vi "IO.vi"() -> ()   [LabVIEW 2020]
uses:
  Global_Variable/Global.vi
  Libraries/S7/S7.lvlib
panel:
  in  "选项卡控件":enum32{"DI", "DO", "伺服"}(tab)
  out "I 1":T1
  out "I 3":T2
  out "I 2":T3
  out "I 0":T4
  out "I 4":T5
  out "I 5":T6
  in  "Q5":T7
  in  "Q4":T8
  in  "Q3":T9
  in  "Q2":T10
  in  "Q1":T11
  in  "Q0":T12
  in  "工位一系数":dbl=1.0
  in  "工位二系数":dbl=1.0
  out "工位一编码器位移":sgl caption="工位一编码器" format="%#.3f"
  out "工位二编码器位移":sgl caption="工位二编码器" format="%#.3f"
  out "工位一扭矩":sgl format="%#.3f"
  out "工位二扭矩":sgl format="%#.3f"
  in  "工位二移载伺服手动速度":sgl caption="手动速度" format="%#.3f"
  in  "工位二移载伺服-正转":bool
  in  "工位二移载伺服-反转":bool
  in  "工位二移载伺服绝对位置":sgl caption="绝对位置" format="%#.3f"
  in  "工位二移载伺服相对位置":sgl caption="相对位置" format="%#.3f"
  out "工位二移载伺服当前位置":sgl caption="当前位置" format="%#.3f"
  in  "工位二移载伺服-绝对定位":bool
  in  "工位二移载伺服-相对定位":bool
  out "工位二移载伺服状态":bool
  in  "工位一旋转伺服手动速度":sgl caption="手动速度" format="%#.3f"
  in  "工位一旋转伺服-正转":bool
  in  "工位一旋转伺服-反转":bool
  in  "工位一旋转伺服绝对位置":sgl caption="绝对位置" format="%#.3f"
  in  "工位一旋转伺服相对位置":sgl caption="相对位置" format="%#.3f"
  out "工位一驱动伺服当前位置":sgl caption="当前位置" format="%#.3f"
  in  "工位一旋转伺服-绝对定位":bool
  in  "工位一旋转伺服-相对定位":bool
  in  "工位二旋转伺服手动速度":sgl caption="手动速度" format="%#.3f"
  in  "工位二旋转伺服-正转":bool
  in  "工位二旋转伺服-反转":bool
  in  "工位二旋转伺服绝对位置":sgl caption="绝对位置" format="%#.3f"
  in  "工位二旋转伺服相对位置":sgl caption="相对位置" format="%#.3f"
  out "工位二驱动伺服当前位置":sgl caption="当前位置" format="%#.3f"
  in  "工位二旋转伺服-绝对定位":bool
  in  "工位二旋转伺服-相对定位":bool
  in  "工位一移载伺服手动速度":sgl caption="手动速度" format="%#.3f"
  in  "工位一移载伺服-正转":bool
  in  "工位一移载伺服-反转":bool
  in  "工位一移载伺服绝对位置":sgl caption="绝对位置" format="%#.3f"
  in  "工位一移载伺服相对位置":sgl caption="相对位置" format="%#.3f"
  out "工位一移载当前位置":sgl caption="当前位置" format="%#.3f"
  in  "工位一移载伺服-绝对定位":bool
  in  "工位一移载伺服-相对定位":bool
  out "工位一旋转伺服状态":bool
  out "工位二旋转伺服状态":bool
  out "工位一移载伺服状态":bool
  # "手动操作"
  # "工位二移载伺服"
  # "工位一旋转伺服"
  # "工位一移载伺服"
  # "工位二旋转伺服"
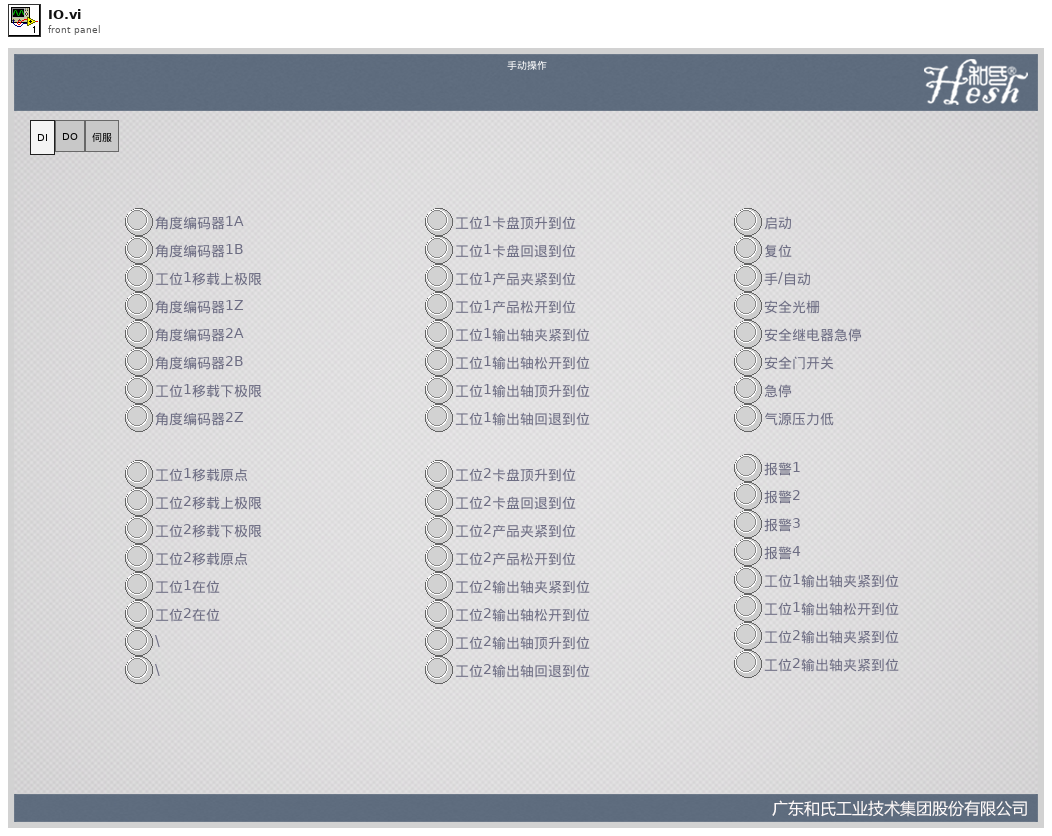
[diagram p1: front panel]
types:
  T1 = cluster{"工位1移载原点":bool, "工位2移载上极限":bool, "工位2移载下极限":bool, "工位2移载原点":bool, "工位1在位":bool, "工位2在位":bool, "\\":bool, "\\ ":bool}
  T2 = cluster{"工位2卡盘顶升到位":bool, "工位2卡盘回退到位":bool, "工位2产品夹紧到位":bool, "工位2产品松开到位":bool, "工位2输出轴夹紧到位":bool, "工位2输出轴松开到位":bool, "工位2输出轴顶升到位":bool, "工位2输出轴回退到位":bool}
  T3 = cluster{"工位1卡盘顶升到位":bool, "工位1卡盘回退到位":bool, "工位1产品夹紧到位":bool, "工位1产品松开到位":bool, "工位1输出轴夹紧到位":bool, "工位1输出轴松开到位":bool, "工位1输出轴顶升到位":bool, "工位1输出轴回退到位":bool}
  T4 = cluster{"角度编码器1A":bool, "角度编码器1B":bool, "工位1移载上极限":bool, "角度编码器1Z":bool, "角度编码器2A":bool, "角度编码器2B":bool, "工位1移载下极限":bool, "角度编码器2Z":bool}
  T5 = cluster{"启动":bool, "复位":bool, "手/自动":bool, "安全光栅":bool, "安全继电器急停":bool, "安全门开关":bool, "急停":bool, "气源压力低":bool}
  T6 = cluster{"报警1":bool, "报警2":bool, "报警3":bool, "报警4":bool, "工位1输出轴夹紧到位":bool, "工位1输出轴松开到位":bool, "工位2输出轴夹紧到位":bool, "工位2输出轴夹紧到位":bool}
  T7 = cluster{"工位1卡盘顶升":bool, "工位1卡盘回退":bool, "工位2卡盘顶升":bool, "工位2卡盘回退":bool, "备用":bool, "备用":bool, "备用":bool, "备用":bool}
  T8 = cluster{"工位1合格指示灯":bool, "工位1不合格指示灯":bool, "工位2合格指示灯":bool, "工位2不合格指示灯":bool, "总气阀":bool, "工位2采集切换":bool, "工位1采集切换":bool, "备用":bool}
  T9 = cluster{"工位2输入轴夹紧":bool, "工位2输入轴松开":bool, "工位2产品夹紧":bool, "工位2产品松开":bool, "工位2输出轴夹紧":bool, "工位2输出轴松开":bool, "工位2输出轴顶升":bool, "工位2输出轴回退":bool}
  T10 = cluster{"工位1输入轴夹紧":bool, "工位1输入轴松开":bool, "工位1产品夹紧":bool, "工位1产品松开":bool, "工位1输出轴夹紧":bool, "工位1输出轴松开":bool, "工位1输出轴顶升":bool, "工位1输出轴回退":bool}
  T11 = cluster{"备用":bool, "备用":bool, "/":bool, "/":bool, "/":bool, "/":bool, "/":bool, "/":bool}
  T12 = cluster{"备用":bool, "备用":bool, "备用":bool, "备用":bool, "三色灯-红":bool, "三色灯-黄":bool, "三色灯-绿":bool, "三色灯-蜂鸣器":bool}
  T13 = cluster{bool, bool, bool, bool, bool, bool, bool, bool}
  T14 = typedef "S7.lvlib/Read_Data (Reply Payload)--cluster.ctl" = cluster{"读取成功":bool, "数据":u32[], "Read_Data_error":errorcluster}
  T15 = cluster{"Boolean array[0]":bool, "Boolean array[1]":bool, "Boolean array[2]":bool, "Boolean array[3]":bool, "Boolean array[4]":bool, "Boolean array[5]":bool, "Boolean array[6]":bool, "Boolean array[7]":bool}
  T16 = cluster{"工位一驱动伺服位移":sgl, "工位二驱动伺服位移":sgl, "工位一移载伺服位移":sgl, "工位二移载伺服位移":sgl, "工位一编码器位移":sgl, "工位二编码器位移":sgl, "工位一扭矩":sgl, "工位二扭矩":sgl}
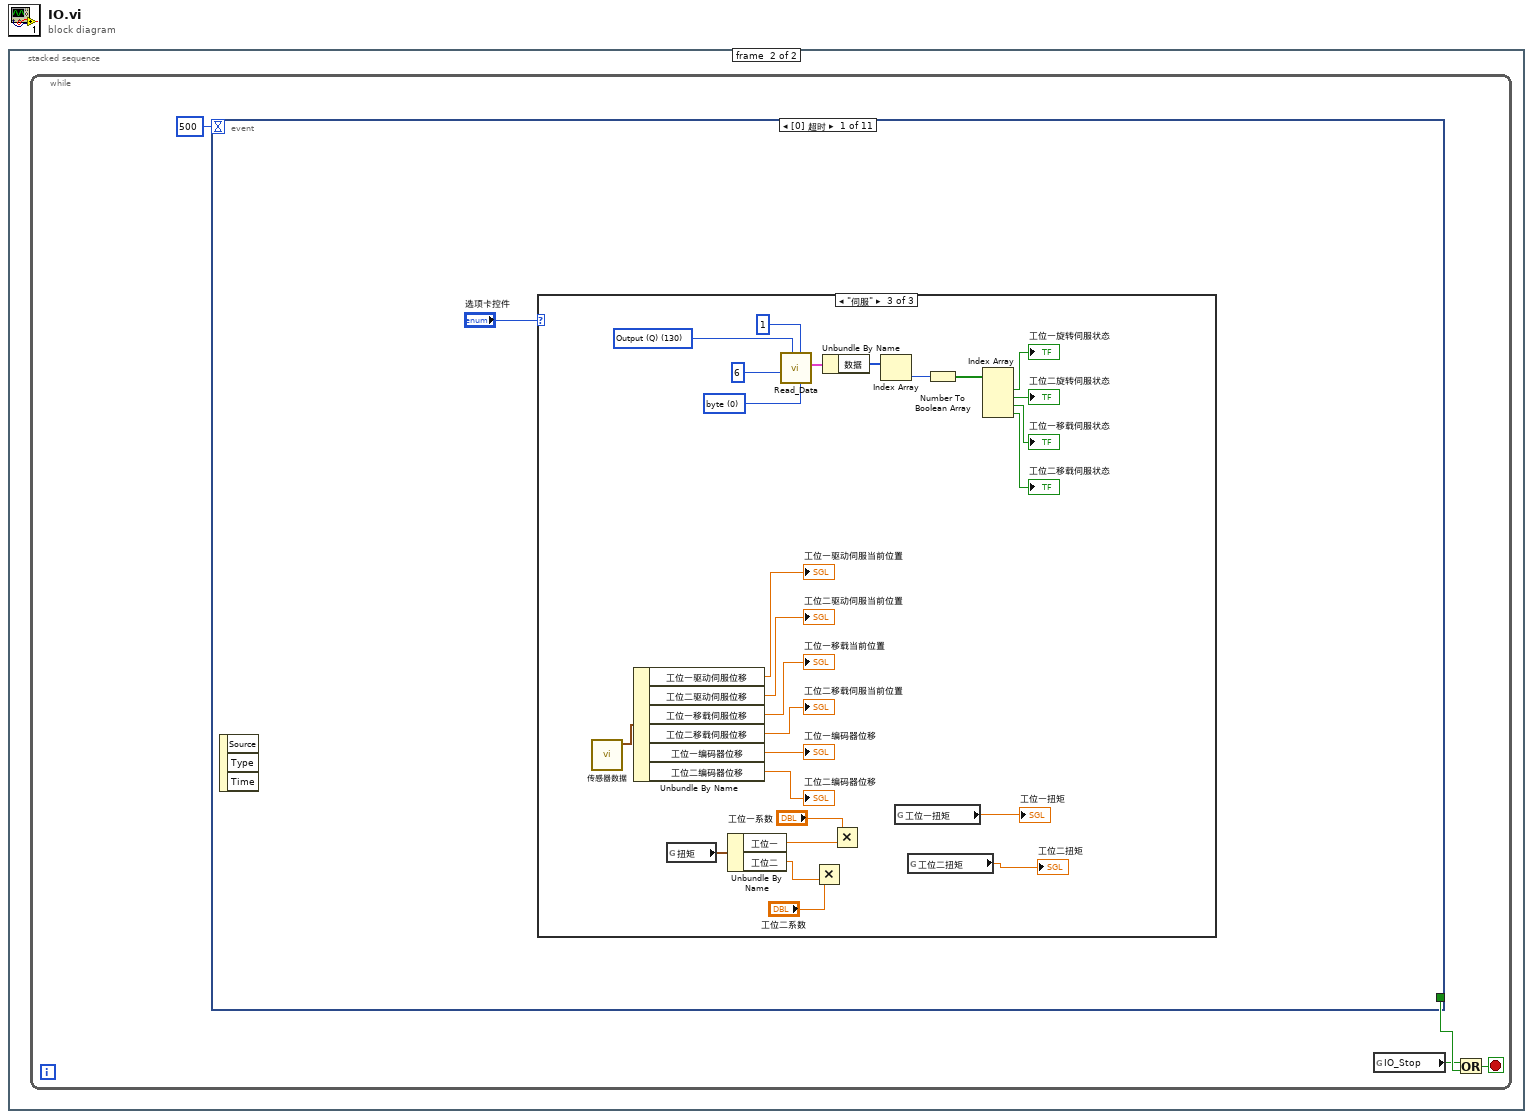
[diagram p0: block diagram]
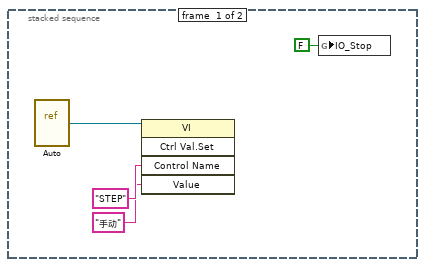
[diagram p2: hidden frame]
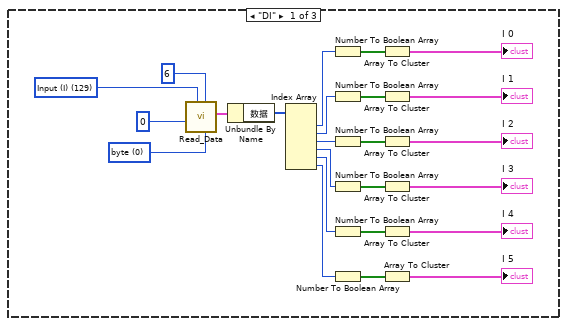
[diagram p3: hidden frame]
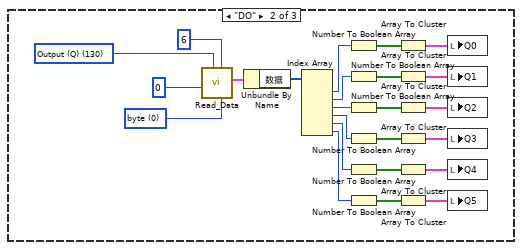
[diagram p4: hidden frame]
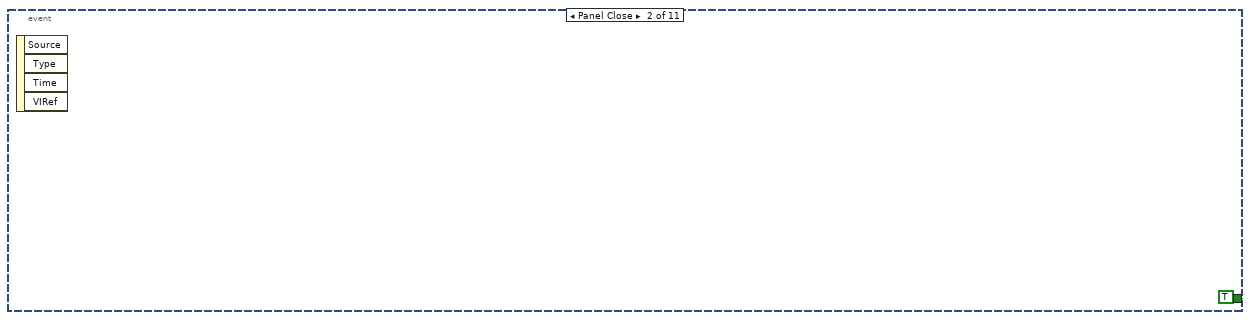
[diagram p5: hidden frame]
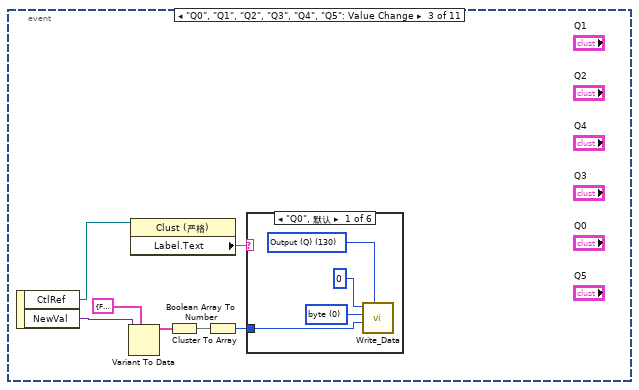
[diagram p6: hidden frame]
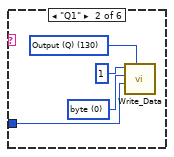
[diagram p7: hidden frame]
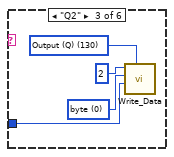
[diagram p8: hidden frame]
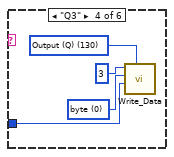
[diagram p9: hidden frame]
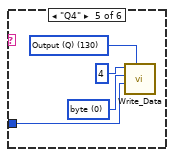
[diagram p10: hidden frame]
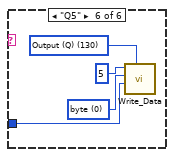
[diagram p11: hidden frame]
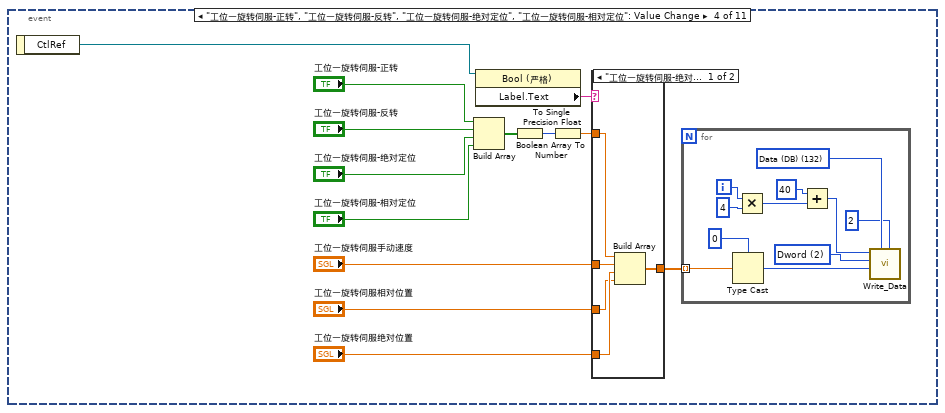
[diagram p12: hidden frame]
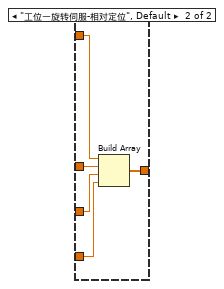
[diagram p13: hidden frame]
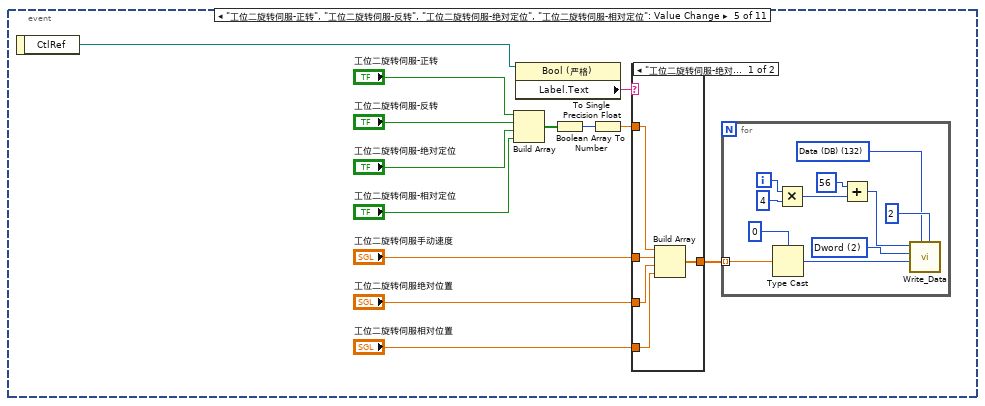
[diagram p14: hidden frame]
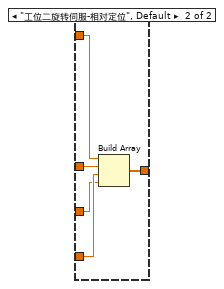
[diagram p15: hidden frame]
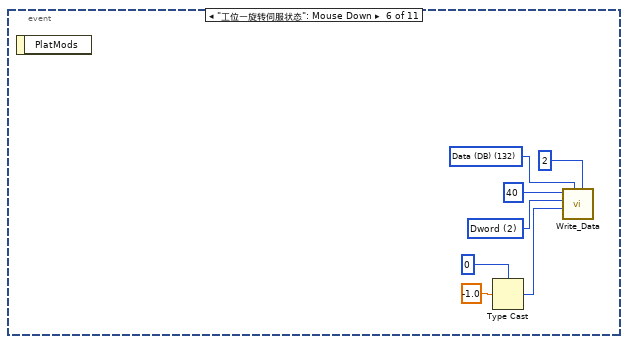
[diagram p16: hidden frame]
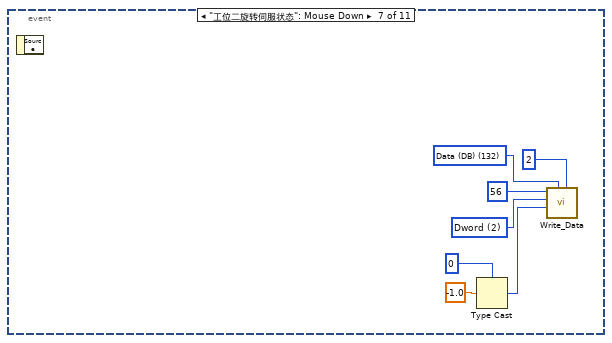
[diagram p17: hidden frame]
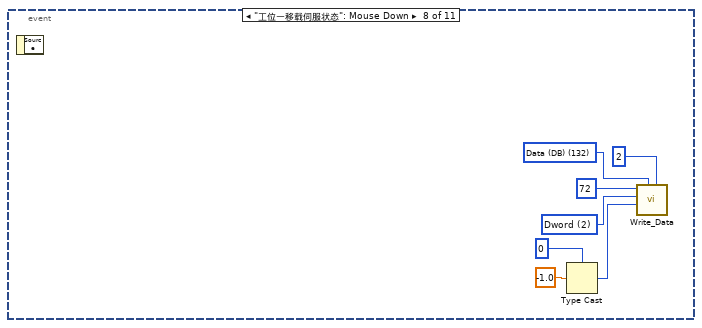
[diagram p18: hidden frame]
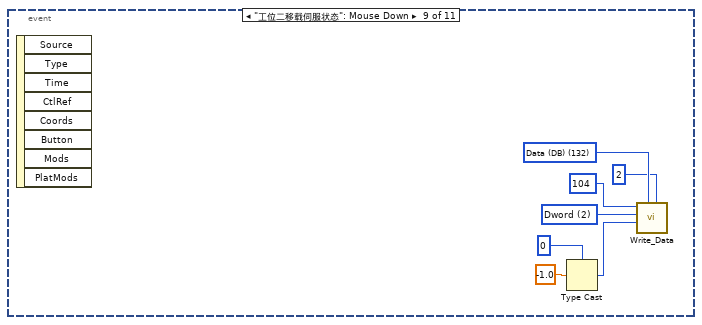
[diagram p19: hidden frame]
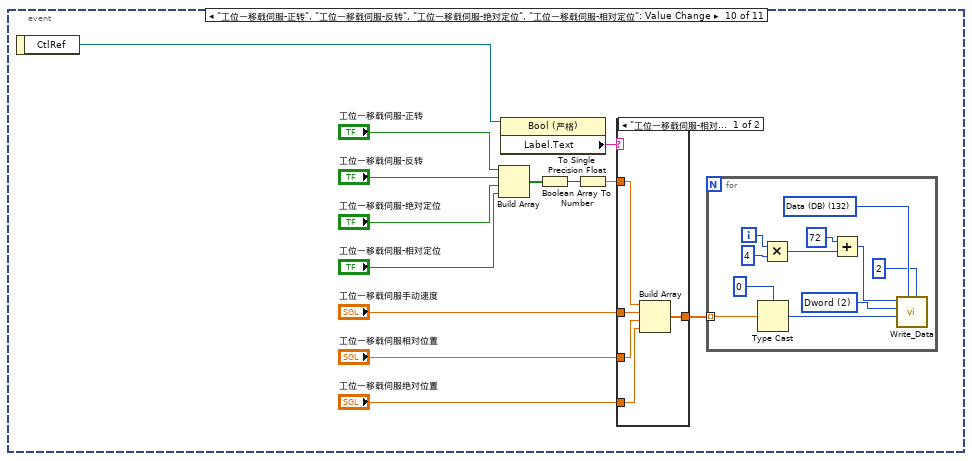
[diagram p20: hidden frame]
diagram:
  n1 = stacked-sequence {
    frame #0 {
      n2 = vi-ref "Auto.vi"() -> (w3:refnum<vi>)
      n3 = invoke class="VI" method="Ctrl Val.Set"(reference=w3, "Control Name"="STEP" ("控件名"), "Value"="手动" ("控件名")) -> ()  [unwired: 2 in, 5 out]
      n4 = global write "Global.vi" "IO_Stop"(FALSE ("IO_Stop")) -> ()
    }
    frame #1 {
      n5 = while {
        stop <- w5 stop-if-true
        n6 = event shown="[0] 超时" {
          selector: _ -> [_ _ _ _ _ _ _ _ _ _ _]
          dyn-events: _ -> [_ _ _ _ _ _ _ _ _ _ _]
          timeout: 500 -> [_ _ _ _ _ _ _ _ _ _ _]
          tunnel: [_ TRUE _ _ _ _ _ _ _ _ _] -> w7
          event Timeout {
            n7 = event-data() -> ()  [unwired: 1 in, 3 out]
            n8 = case shown="\"伺服\"" "选项卡控件" {
              frame "DI" {
                w13 = u16 0 items=["byte", "word", "Dword"] ("数据类型")
                w11 = u8 129 items=["I/O (P)"=128, "Input (I)"=129, "Output (Q)"=130, "Bit Memory (M)"=131, "Data (DB)"=132, "Instance Data (DI)"=133, "Local Data (L)"=134, "Predecessor Local Data (VL)"=135] ("寄存器类型")
                n9 = call "Read_Data.vi"("数据类型"=w13, "读取长度"=u16 6, "寄存器类型"=w11, "起始地址"=u32 0) -> ("Reply Payload"=w15:T14)  [unwired: 5 in, 2 out]
                n10 = Unbundle By Name(w15) -> ("数据"=w14:u32[])
                n11 = Index Array(array=w14) -> (element #1=w27:u32, element #2=w29:u32, element #3=w28:u32, element #4=w24:u32, element #5=w23:u32, element #6=w22:u32)  [unwired: 6 in]
                n12 = Number To Boolean Array(number=w27) -> (Boolean array=w26:bool[])
                n13 = Number To Boolean Array(number=w29) -> (Boolean array=w25:bool[])
                n14 = Number To Boolean Array(number=w28) -> (Boolean array=w21:bool[])
                n15 = Number To Boolean Array(number=w24) -> (Boolean array=w19:bool[])
                n16 = Number To Boolean Array(number=w23) -> (Boolean array=w17:bool[])
                n17 = Number To Boolean Array(number=w22) -> (Boolean array=w16:bool[])
                n18 = Array To Cluster(array=w26) -> (cluster=→"I 0":T15)
                n19 = Array To Cluster(array=w25) -> (cluster=→"I 1":T15)
                n20 = Array To Cluster(array=w21) -> (cluster=→"I 2":T15)
                n21 = Array To Cluster(array=w19) -> (cluster=→"I 3":T15)
                n22 = Array To Cluster(array=w17) -> (cluster=→"I 4":T15)
                n23 = Array To Cluster(array=w16) -> (cluster=→"I 5":T15)
              }
              frame "DO" {
                w37 = u16 0 items=["byte", "word", "Dword"] ("数据类型")
                w35 = u8 130 items=["I/O (P)"=128, "Input (I)"=129, "Output (Q)"=130, "Bit Memory (M)"=131, "Data (DB)"=132, "Instance Data (DI)"=133, "Local Data (L)"=134, "Predecessor Local Data (VL)"=135] ("寄存器类型")
                n24 = call "Read_Data.vi"("数据类型"=w37, "读取长度"=u16 6, "寄存器类型"=w35, "起始地址"=u32 0) -> ("Reply Payload"=w56:T14)  [unwired: 5 in, 2 out]
                n25 = Unbundle By Name(w56) -> ("数据"=w57:u32[])
                n26 = Index Array(array=w57) -> (element #1=w47:u32, element #2=w49:u32, element #3=w48:u32, element #4=w46:u32, element #5=w45:u32, element #6=w44:u32)  [unwired: 6 in]
                n27 = Number To Boolean Array(number=w47) -> (Boolean array=w50:bool[])
                n28 = Number To Boolean Array(number=w49) -> (Boolean array=w51:bool[])
                n29 = Number To Boolean Array(number=w48) -> (Boolean array=w52:bool[])
                n30 = Number To Boolean Array(number=w46) -> (Boolean array=w53:bool[])
                n31 = Number To Boolean Array(number=w45) -> (Boolean array=w54:bool[])
                n32 = Number To Boolean Array(number=w44) -> (Boolean array=w55:bool[])
                n33 = Array To Cluster(array=w50) -> (cluster=w42:T15)
                n34 = Array To Cluster(array=w51) -> (cluster=w43:T15)
                n35 = Array To Cluster(array=w52) -> (cluster=w40:T15)
                n36 = Array To Cluster(array=w53) -> (cluster=w41:T15)
                n37 = Array To Cluster(array=w54) -> (cluster=w39:T15)
                n38 = Array To Cluster(array=w55) -> (cluster=w38:T15)
                n39 = local write "Q0"(w42) -> ()
                n40 = local write "Q1"(w43) -> ()
                n41 = local write "Q2"(w40) -> ()
                n42 = local write "Q3"(w41) -> ()
                n43 = local write "Q4"(w39) -> ()
                n44 = local write "Q5"(w38) -> ()
              }
              frame "伺服" {
                w76 = u16 0 items=["byte", "word", "Dword"] ("数据类型")
                w74 = u8 130 items=["I/O (P)"=128, "Input (I)"=129, "Output (Q)"=130, "Bit Memory (M)"=131, "Data (DB)"=132, "Instance Data (DI)"=133, "Local Data (L)"=134, "Predecessor Local Data (VL)"=135] ("寄存器类型")
                n45 = call "传感器数据.vi"() -> ("传感器读数"=w72:T16)  [unwired: 11 in]
                n46 = Unbundle By Name(w72) -> ("工位一驱动伺服位移"=→"工位一驱动伺服当前位置":sgl, "工位二驱动伺服位移"=→"工位二驱动伺服当前位置":sgl, "工位一移载伺服位移"=→"工位一移载当前位置":sgl, "工位二移载伺服位移"=→"工位二移载伺服当前位置":sgl, "工位一编码器位移"=→"工位一编码器位移":sgl, "工位二编码器位移"=→"工位二编码器位移":sgl)
                n47 = global read "Global.vi" "扭矩"() -> (w64:cluster{"工位一":dbl, "工位二":dbl})
                n48 = Unbundle By Name(w64) -> ("工位一"=w63:dbl, "工位二"=w62:dbl)
                n49 = call "Read_Data.vi"("数据类型"=w76, "读取长度"=u16 1, "寄存器类型"=w74, "起始地址"=u32 6) -> ("Reply Payload"=w77:T14)  [unwired: 5 in, 2 out]
                n50 = Multiply(x="工位二系数", y=w62) -> ()  [unwired: 1 out]
                n51 = Unbundle By Name(w77) -> ("数据"=w78:u32[])
                n52 = Multiply(x="工位一系数", y=w63) -> ()  [unwired: 1 out]
                n53 = Index Array(array=w78) -> (element=w83:u32)  [unwired: 1 in]
                n54 = global read "Global.vi" "工位一扭矩"() -> (→"工位一扭矩":dbl)
                n55 = global read "Global.vi" "工位二扭矩"() -> (→"工位二扭矩":dbl)
                n56 = Number To Boolean Array(number=w83) -> (Boolean array=w80:bool[])
                n57 = Index Array(array=w80) -> (element #1=→"工位一旋转伺服状态":bool, element #2=→"工位二旋转伺服状态":bool, element #3=→"工位一移载伺服状态":bool, element #4=→"工位二移载伺服状态":bool)  [unwired: 4 in]
              }
            }
          }
          event Panel Close {
            n58 = event-data() -> ()  [unwired: 1 in, 4 out]
          }
          event "Q0", "Q1", "Q2", "Q3", "Q4", "Q5": Value Change {
            n59 = event-data() -> ("CtlRef"=w86:refnum<vi>, "NewVal"=w90:variant)  [unwired: 1 in]
            n60 = Variant To Data(type=T13 {FALSE, FALSE, FALSE, FALSE, FALSE, FALSE, FALSE, FALSE}, Variant=w90) -> (data=w89:T13)  [unwired: 1 in, 1 out]
            n61 = property class="Clust (严格)"(reference=w86) -> ("Label.Text"=w85:string)  [unwired: 1 in, 2 out]
            n62 = Cluster To Array(cluster=w89) -> (array=w88:bool[])
            n63 = Boolean Array To Number(Boolean array=w88) -> (number=w87:u32)
            n64 = case shown="\"Q0\", 默认" w85 {
              tunnel: w87 -> [w95 w99 w103 w107 w111 w115]
              frame "Q0", Default {
                w93 = u16 0 items=["byte", "word", "Dword"] ("数据类型")
                w94 = u8 130 items=["I/O (P)"=128, "Input (I)"=129, "Output (Q)"=130, "Bit Memory (M)"=131, "Data (DB)"=132, "Instance Data (DI)"=133, "Local Data (L)"=134, "Predecessor Local Data (VL)"=135] ("寄存器类型")
                n65 = call "Write_Data.vi"("寄存器类型"=w94, "写入数据"=w95, "数据类型"=w93, "写入地址"=u32 0) -> ()  [unwired: 5 in, 3 out]
              }
              frame "Q1" {
                w97 = u16 0 items=["byte", "word", "Dword"] ("数据类型")
                w98 = u8 130 items=["I/O (P)"=128, "Input (I)"=129, "Output (Q)"=130, "Bit Memory (M)"=131, "Data (DB)"=132, "Instance Data (DI)"=133, "Local Data (L)"=134, "Predecessor Local Data (VL)"=135] ("寄存器类型")
                n66 = call "Write_Data.vi"("寄存器类型"=w98, "写入数据"=w99, "数据类型"=w97, "写入地址"=u32 1) -> ()  [unwired: 5 in, 3 out]
              }
              frame "Q2" {
                w101 = u16 0 items=["byte", "word", "Dword"] ("数据类型")
                w102 = u8 130 items=["I/O (P)"=128, "Input (I)"=129, "Output (Q)"=130, "Bit Memory (M)"=131, "Data (DB)"=132, "Instance Data (DI)"=133, "Local Data (L)"=134, "Predecessor Local Data (VL)"=135] ("寄存器类型")
                n67 = call "Write_Data.vi"("寄存器类型"=w102, "写入数据"=w103, "数据类型"=w101, "写入地址"=u32 2) -> ()  [unwired: 5 in, 3 out]
              }
              frame "Q3" {
                w105 = u16 0 items=["byte", "word", "Dword"] ("数据类型")
                w106 = u8 130 items=["I/O (P)"=128, "Input (I)"=129, "Output (Q)"=130, "Bit Memory (M)"=131, "Data (DB)"=132, "Instance Data (DI)"=133, "Local Data (L)"=134, "Predecessor Local Data (VL)"=135] ("寄存器类型")
                n68 = call "Write_Data.vi"("寄存器类型"=w106, "写入数据"=w107, "数据类型"=w105, "写入地址"=u32 3) -> ()  [unwired: 5 in, 3 out]
              }
              frame "Q4" {
                w109 = u16 0 items=["byte", "word", "Dword"] ("数据类型")
                w110 = u8 130 items=["I/O (P)"=128, "Input (I)"=129, "Output (Q)"=130, "Bit Memory (M)"=131, "Data (DB)"=132, "Instance Data (DI)"=133, "Local Data (L)"=134, "Predecessor Local Data (VL)"=135] ("寄存器类型")
                n69 = call "Write_Data.vi"("寄存器类型"=w110, "写入数据"=w111, "数据类型"=w109, "写入地址"=u32 4) -> ()  [unwired: 5 in, 3 out]
              }
              frame "Q5" {
                w113 = u16 0 items=["byte", "word", "Dword"] ("数据类型")
                w114 = u8 130 items=["I/O (P)"=128, "Input (I)"=129, "Output (Q)"=130, "Bit Memory (M)"=131, "Data (DB)"=132, "Instance Data (DI)"=133, "Local Data (L)"=134, "Predecessor Local Data (VL)"=135] ("寄存器类型")
                n70 = call "Write_Data.vi"("寄存器类型"=w114, "写入数据"=w115, "数据类型"=w113, "写入地址"=u32 5) -> ()  [unwired: 5 in, 3 out]
              }
            }
          }
          event "工位一旋转伺服-正转", "工位一旋转伺服-反转", "工位一旋转伺服-绝对定位", "工位一旋转伺服-相对定位": Value Change {
            n71 = event-data() -> ("CtlRef"=w128:refnum<vi>)  [unwired: 1 in]
            n72 = Build Array("工位一旋转伺服-正转", "工位一旋转伺服-反转", "工位一旋转伺服-绝对定位", "工位一旋转伺服-相对定位") -> (w121:bool[])
            n73 = property class="Bool (严格)"(reference=w128) -> ("Label.Text"=w127:string)  [unwired: 1 in, 2 out]
            n74 = Boolean Array To Number(Boolean array=w121) -> (number=w122:u32)
            n75 = To Single Precision Float(number=w122) -> (single precision float=w120:sgl)
            n76 = case shown="\"工位一旋转伺服-绝对定位\"" w127 {
              tunnel: w120 -> [w144 w149]
              tunnel: "工位一旋转伺服相对位置" -> [w140 w148]
              tunnel: "工位一旋转伺服绝对位置" -> [w141 w147]
              tunnel: "工位一旋转伺服手动速度" -> [w143 w146]
              tunnel: [w142 w145] -> w116
              frame "工位一旋转伺服-绝对定位" {
                n77 = Build Array(w144, w143, w141, w140) -> (w142:sgl[])
              }
              frame "工位一旋转伺服-相对定位", Default {
                n78 = Build Array(w149, w146, w148, w147) -> (w145:sgl[])
              }
            }
            n79 = for {
              tunnel: w116 -> [w134] mode=indexing
              i -> [w131]
              w136 = u16 2 items=["byte", "word", "Dword"] ("数据类型")
              w139 = u8 132 items=["I/O (P)"=128, "Input (I)"=129, "Output (Q)"=130, "Bit Memory (M)"=131, "Data (DB)"=132, "Instance Data (DI)"=133, "Local Data (L)"=134, "Predecessor Local Data (VL)"=135] ("寄存器类型")
              n80 = Type Cast(type=u32 0, x=w134) -> (*(type *) &x=w133:u32)
              n81 = Multiply(x=w131, y=u32 4) -> (x*y=w130:u32)
              n82 = Add(x=u32 40 ("写入地址"), y=w130) -> (x+y=w129:u32)
              n83 = call "Write_Data.vi"("DB #"=u16 2, "寄存器类型"=w139, "写入数据"=w133, "数据类型"=w136, "写入地址"=w129) -> ()  [unwired: 4 in, 3 out]
            }
          }
          event "工位二旋转伺服-正转", "工位二旋转伺服-反转", "工位二旋转伺服-绝对定位", "工位二旋转伺服-相对定位": Value Change {
            n84 = event-data() -> ("CtlRef"=w151:refnum<vi>)  [unwired: 1 in]
            n85 = Build Array("工位二旋转伺服-正转", "工位二旋转伺服-反转", "工位二旋转伺服-绝对定位", "工位二旋转伺服-相对定位") -> (w161:bool[])
            n86 = property class="Bool (严格)"(reference=w151) -> ("Label.Text"=w150:string)  [unwired: 1 in, 2 out]
            n87 = Boolean Array To Number(Boolean array=w161) -> (number=w160:u32)
            n88 = To Single Precision Float(number=w160) -> (single precision float=w162:sgl)
            n89 = case shown="\"工位二旋转伺服-绝对定位\"" w150 {
              tunnel: w162 -> [w167 w172]
              tunnel: [w166 w171] -> w159
              tunnel: "工位二旋转伺服手动速度" -> [w165 w170]
              tunnel: "工位二旋转伺服相对位置" -> [w163 w169]
              tunnel: "工位二旋转伺服绝对位置" -> [w164 w168]
              frame "工位二旋转伺服-绝对定位" {
                n90 = Build Array(w167, w165, w164, w163) -> (w166:sgl[])
              }
              frame "工位二旋转伺服-相对定位", Default {
                n91 = Build Array(w172, w170, w169, w168) -> (w171:sgl[])
              }
            }
            n92 = for {
              tunnel: w159 -> [w181] mode=indexing
              i -> [w179]
              w174 = u16 2 items=["byte", "word", "Dword"] ("数据类型")
              w176 = u8 132 items=["I/O (P)"=128, "Input (I)"=129, "Output (Q)"=130, "Bit Memory (M)"=131, "Data (DB)"=132, "Instance Data (DI)"=133, "Local Data (L)"=134, "Predecessor Local Data (VL)"=135] ("寄存器类型")
              n93 = Type Cast(type=u32 0, x=w181) -> (*(type *) &x=w173:u32)
              n94 = Multiply(x=w179, y=u32 4) -> (x*y=w178:u32)
              n95 = Add(x=u32 56 ("写入地址"), y=w178) -> (x+y=w175:u32)
              n96 = call "Write_Data.vi"("DB #"=u16 2, "寄存器类型"=w176, "写入数据"=w173, "数据类型"=w174, "写入地址"=w175) -> ()  [unwired: 4 in, 3 out]
            }
          }
          event "工位一旋转伺服状态": Mouse Down {
            w186 = u16 2 items=["byte", "word", "Dword"] ("数据类型")
            w188 = u8 132 items=["I/O (P)"=128, "Input (I)"=129, "Output (Q)"=130, "Bit Memory (M)"=131, "Data (DB)"=132, "Instance Data (DI)"=133, "Local Data (L)"=134, "Predecessor Local Data (VL)"=135] ("寄存器类型")
            n97 = event-data() -> ()  [unwired: 1 in, 1 out]
            n98 = Type Cast(type=u32 0, x=sgl -1.0) -> (*(type *) &x=w190:u32)
            n99 = call "Write_Data.vi"("DB #"=u16 2, "寄存器类型"=w188, "写入数据"=w190, "数据类型"=w186, "写入地址"=u32 40) -> ()  [unwired: 4 in, 3 out]
          }
          event "工位二旋转伺服状态": Mouse Down {
            w191 = u16 2 items=["byte", "word", "Dword"] ("数据类型")
            w194 = u8 132 items=["I/O (P)"=128, "Input (I)"=129, "Output (Q)"=130, "Bit Memory (M)"=131, "Data (DB)"=132, "Instance Data (DI)"=133, "Local Data (L)"=134, "Predecessor Local Data (VL)"=135] ("寄存器类型")
            n100 = event-data() -> ()  [unwired: 1 in, 1 out]
            n101 = Type Cast(type=u32 0, x=sgl -1.0) -> (*(type *) &x=w197:u32)
            n102 = call "Write_Data.vi"("DB #"=u16 2, "寄存器类型"=w194, "写入数据"=w197, "数据类型"=w191, "写入地址"=u32 56) -> ()  [unwired: 4 in, 3 out]
          }
          event "工位一移载伺服状态": Mouse Down {
            w198 = u16 2 items=["byte", "word", "Dword"] ("数据类型")
            w201 = u8 132 items=["I/O (P)"=128, "Input (I)"=129, "Output (Q)"=130, "Bit Memory (M)"=131, "Data (DB)"=132, "Instance Data (DI)"=133, "Local Data (L)"=134, "Predecessor Local Data (VL)"=135] ("寄存器类型")
            n103 = event-data() -> ()  [unwired: 1 in, 1 out]
            n104 = Type Cast(type=u32 0, x=sgl -1.0) -> (*(type *) &x=w204:u32)
            n105 = call "Write_Data.vi"("DB #"=u16 2, "寄存器类型"=w201, "写入数据"=w204, "数据类型"=w198, "写入地址"=u32 72) -> ()  [unwired: 4 in, 3 out]
          }
          event "工位二移载伺服状态": Mouse Down {
            w205 = u16 2 items=["byte", "word", "Dword"] ("数据类型")
            w208 = u8 132 items=["I/O (P)"=128, "Input (I)"=129, "Output (Q)"=130, "Bit Memory (M)"=131, "Data (DB)"=132, "Instance Data (DI)"=133, "Local Data (L)"=134, "Predecessor Local Data (VL)"=135] ("寄存器类型")
            n106 = event-data() -> ()  [unwired: 1 in, 8 out]
            n107 = Type Cast(type=u32 0, x=sgl -1.0) -> (*(type *) &x=w211:u32)
            n108 = call "Write_Data.vi"("DB #"=u16 2, "寄存器类型"=w208, "写入数据"=w211, "数据类型"=w205, "写入地址"=u32 104) -> ()  [unwired: 4 in, 3 out]
          }
          event "工位一移载伺服-正转", "工位一移载伺服-反转", "工位一移载伺服-绝对定位", "工位一移载伺服-相对定位": Value Change {
            n109 = event-data() -> ("CtlRef"=w213:refnum<vi>)  [unwired: 1 in]
            n110 = Build Array("工位一移载伺服-正转", "工位一移载伺服-反转", "工位一移载伺服-绝对定位", "工位一移载伺服-相对定位") -> (w220:bool[])
            n111 = property class="Bool (严格)"(reference=w213) -> ("Label.Text"=w212:string)  [unwired: 1 in, 2 out]
            n112 = Boolean Array To Number(Boolean array=w220) -> (number=w219:u32)
            n113 = To Single Precision Float(number=w219) -> (single precision float=w218:sgl)
            n114 = case shown="\"工位一移载伺服-相对定位 \", 默认" w212 {
              tunnel: w218 -> [w229 w234]
              tunnel: "工位一移载伺服手动速度" -> [w228 w233]
              tunnel: [w227 w232] -> w216
              tunnel: "工位一移载伺服绝对位置" -> [w226 w230]
              tunnel: "工位一移载伺服相对位置" -> [w225 w231]
              frame "工位一移载伺服-相对定位 ", Default {
                n115 = Build Array(w229, w228, w225, w226) -> (w227:sgl[])
              }
              frame "工位一移载伺服-绝对定位" {
                n116 = Build Array(w234, w233, w230, w231) -> (w232:sgl[])
              }
            }
            n117 = for {
              tunnel: w216 -> [w240] mode=indexing
              i -> [w237]
              w242 = u16 2 items=["byte", "word", "Dword"] ("数据类型")
              w245 = u8 132 items=["I/O (P)"=128, "Input (I)"=129, "Output (Q)"=130, "Bit Memory (M)"=131, "Data (DB)"=132, "Instance Data (DI)"=133, "Local Data (L)"=134, "Predecessor Local Data (VL)"=135] ("寄存器类型")
              n118 = Type Cast(type=u32 0, x=w240) -> (*(type *) &x=w239:u32)
              n119 = Multiply(x=w237, y=u32 4) -> (x*y=w236:u32)
              n120 = Add(x=u32 72 ("写入地址"), y=w236) -> (x+y=w235:u32)
              n121 = call "Write_Data.vi"("DB #"=u16 2, "寄存器类型"=w245, "写入数据"=w239, "数据类型"=w242, "写入地址"=w235) -> ()  [unwired: 4 in, 3 out]
            }
          }
          event "工位二移载伺服-正转", "工位二移载伺服-反转", "工位二移载伺服-绝对定位", "工位二移载伺服-相对定位": Value Change {
            n122 = event-data() -> ("CtlRef"=w247:refnum<vi>)  [unwired: 1 in]
            n123 = Build Array("工位二移载伺服-正转", "工位二移载伺服-反转", "工位二移载伺服-绝对定位", "工位二移载伺服-相对定位") -> (w251:bool[])
            n124 = property class="Bool (严格)"(reference=w247) -> ("Label.Text"=w246:string)  [unwired: 1 in, 2 out]
            n125 = Boolean Array To Number(Boolean array=w251) -> (number=w250:u32)
            n126 = To Single Precision Float(number=w250) -> (single precision float=w249:sgl)
            n127 = case shown="\"工位二移载伺服-绝对定位\"" w246 {
              tunnel: "工位二移载伺服绝对位置" -> [w263 w265]
              tunnel: "工位二移载伺服相对位置" -> [w262 w264]
              tunnel: "工位二移载伺服手动速度" -> [w261 w268]
              tunnel: w249 -> [w260 w267]
              tunnel: [w259 w266] -> w248
              frame "工位二移载伺服-相对定位", Default {
                n128 = Build Array(w260, w261, w262, w263) -> (w259:sgl[])
              }
              frame "工位二移载伺服-绝对定位" {
                n129 = Build Array(w267, w268, w265, w264) -> (w266:sgl[])
              }
            }
            n130 = for {
              tunnel: w248 -> [w274] mode=indexing
              i -> [w271]
              w276 = u16 2 items=["byte", "word", "Dword"] ("数据类型")
              w279 = u8 132 items=["I/O (P)"=128, "Input (I)"=129, "Output (Q)"=130, "Bit Memory (M)"=131, "Data (DB)"=132, "Instance Data (DI)"=133, "Local Data (L)"=134, "Predecessor Local Data (VL)"=135] ("寄存器类型")
              n131 = Type Cast(type=u32 0, x=w274) -> (*(type *) &x=w273:u32)
              n132 = Multiply(x=w271, y=u32 4) -> (x*y=w270:u32)
              n133 = Add(x=u32 104 ("写入地址"), y=w270) -> (x+y=w269:u32)
              n134 = call "Write_Data.vi"("DB #"=u16 2, "寄存器类型"=w279, "写入数据"=w273, "数据类型"=w276, "写入地址"=w269) -> ()  [unwired: 4 in, 3 out]
            }
          }
        }
        n135 = global read "Global.vi" "IO_Stop"() -> (w6:bool)
        n136 = Or(x=w6, y=w7) -> (x .or. y?=w5:bool)
      }
    }
  }
